vi "Address setting.vi"(7 "Address Cluster out输入":T1={"SPU"=refnum, "MPM"=[], "Port_Count"=0.0, "MPM_Count"=0.0, "SPU_Resource"=[], "USB_Resource"=[], "MPM_Communicater"="", "MPM_Count"=0.0, "MPM_Address"=[], "MPM_Portnumber"=[], "SPU_DeviveID"="", "MPM_communcation_method"=[], "TSL_sweepstartwave"=0.0, "TSL_sweepstopwave"=0.0, "TSL_Address"="", "TSL_Communicater"="", "TSL"=refnum, "tsl_communcation_method"=3, "TSL_Portnumber"=0.0} {"tsl_communcation_method" items=["GPIB", "C232C", "TCPIP", "USB"]; "MPM_communcation_method" items=["GPIB", "C232C", "TCPIP", "USB"]}, 8 "错误输入（无错误）":errorcluster caption="error in", 11 "SPU in":refnum<k24>) -> (0 "error out":errorcluster, 1 "Address Cluster out输出":T1={"SPU"=refnum, "MPM"=[], "Port_Count"=0.0, "MPM_Count"=0.0, "SPU_Resource"=[], "USB_Resource"=[], "MPM_Communicater"="", "MPM_Count"=0.0, "MPM_Address"=[], "MPM_Portnumber"=[], "SPU_DeviveID"="", "MPM_communcation_method"=[], "TSL_sweepstartwave"=0.0, "TSL_sweepstopwave"=0.0, "TSL_Address"="", "TSL_Communicater"="", "TSL"=refnum, "tsl_communcation_method"=3, "TSL_Portnumber"=0.0} {"tsl_communcation_method" items=["GPIB", "C232C", "TCPIP", "USB"]; "MPM_communcation_method" items=["GPIB", "C232C", "TCPIP", "USB"]})   [LabVIEW 2017]
doc: "'----Apply to communication parametere from Instrument setting form"
uses:
  CTL/Address Cluster.ctl
  D:/test/ILSTS/LV_IL_Sample/DLL/InstrumentDLL.dll
  DLL/InstrumentDLL.dll
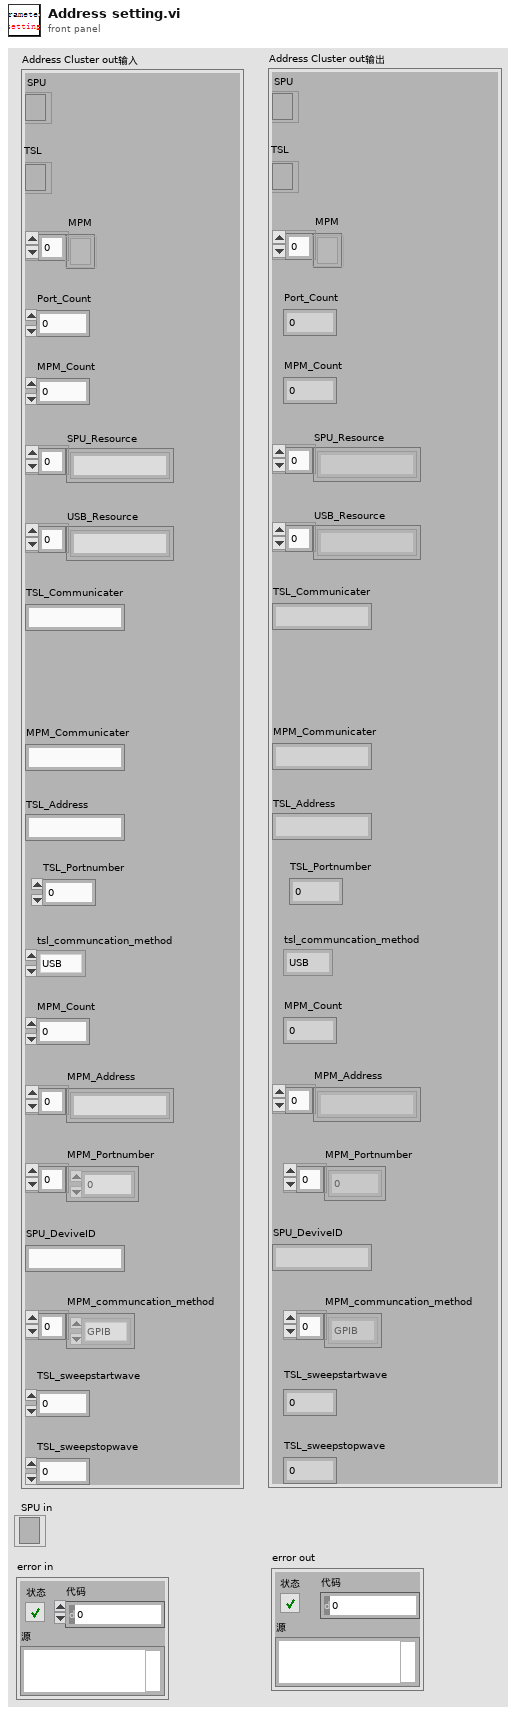
[diagram p1: front panel]
types:
  T1 = typedef "Address Cluster.ctl" = cluster{"SPU":refnum<k24>, "MPM":refnum<k24>[], "Port_Count":dbl, "MPM_Count":dbl, "SPU_Resource":string[], "USB_Resource":string[], "MPM_Communicater":string, "MPM_Count":dbl, "MPM_Address":string[], "MPM_Portnumber":dbl[], "SPU_DeviveID":string, "MPM_communcation_method":i32[], "TSL_sweepstartwave":dbl, "TSL_sweepstopwave":dbl, "TSL_Address":string, "TSL_Communicater":string, "TSL":refnum<k24>, "tsl_communcation_method":i32, "TSL_Portnumber":dbl}
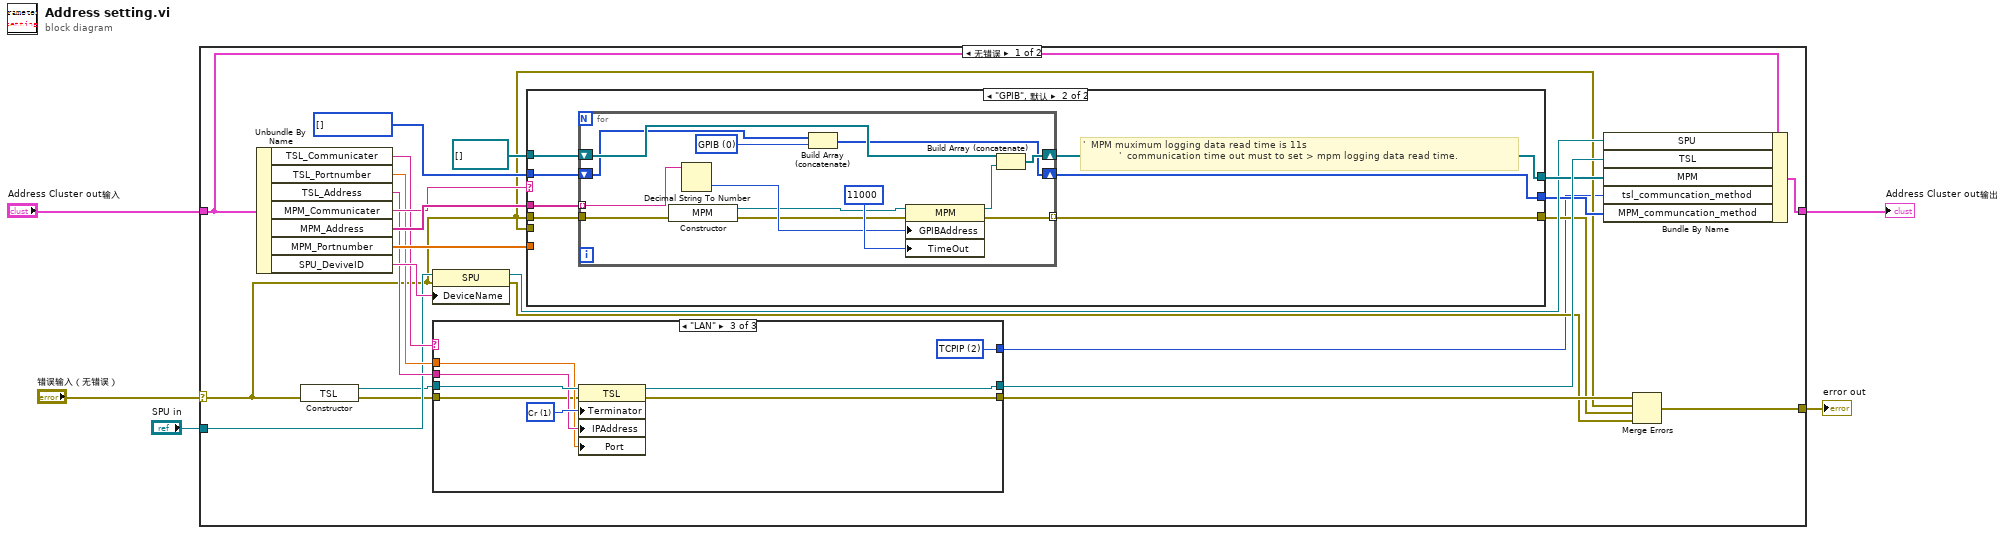
[diagram p0: block diagram]
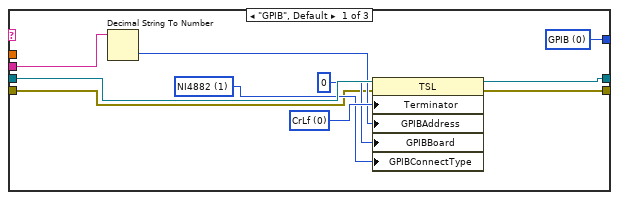
[diagram p2: hidden frame]
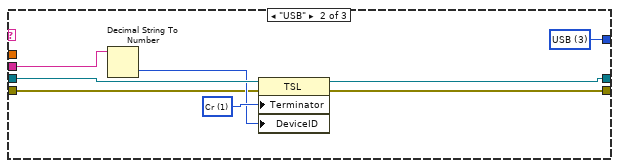
[diagram p3: hidden frame]
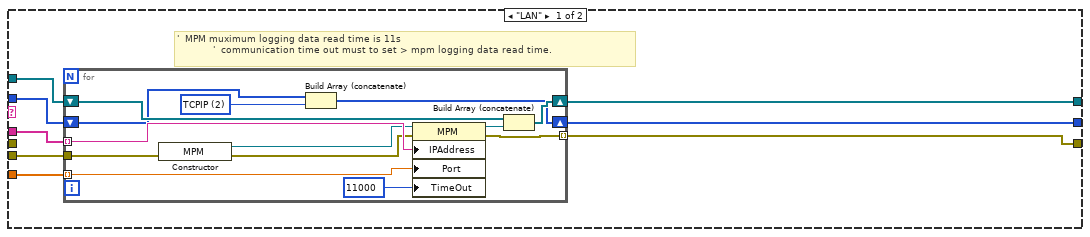
[diagram p4: hidden frame]
diagram:
  n1 = case shown="无错误" "错误输入（无错误）" {
    selector: "错误输入（无错误）" -> [w9 w98]
    tunnel: [w29 w97] -> w5
    tunnel: "Address Cluster out输入" -> [w25 w97]
    tunnel: [w11 w98] -> w3
    tunnel: "SPU in" -> [w10 _]
    frame No Error {
      w23 = i32[] [] items=["GPIB", "C232C", "TCPIP", "USB"] ("tsl_communcation_method")
      n2 = Unbundle By Name(w25) -> ("TSL_Communicater"=w16:string, "TSL_Portnumber"=w18:dbl, "TSL_Address"=w17:string, "MPM_Communicater"=w19:string, "MPM_Address"=w20:string[], "MPM_Portnumber"=w21:dbl[], "SPU_DeviveID"=w24:string)
      n3 = constructor class="TSL"(error in=w9) -> (reference out=w8:refnum<k24>, error out=w7:errorcluster)  [unwired: 2 in, 1 out]
      n4 = property on="属性节点" class="SPU"(reference=w10, error in=w9, "DeviceName"=w24) -> (reference out=w26:refnum<k24>, error out=w12:errorcluster)
      n5 = case shown="\"LAN\"" w16 {
        tunnel: w8 -> [w39 w47 w55]
        tunnel: [w30 w40 w48] -> w28
        tunnel: w17 -> [w37 w45 w53]
        tunnel: w18 -> [_ _ w52]
        tunnel: w7 -> [w33 w43 w51]
        tunnel: [w32 w42 w50] -> w14
        tunnel: [w31 w41 w49] -> w6
        frame "GPIB", Default {
          w34 = 1 items=["NIVisa", "NI4882", "KeysightIO"] ("GPIBConnectType")
          w38 = 0 items=["CrLf", "Cr", "Lf"] ("Terminator")
          w31 = 0 items=["GPIB", "C232C", "TCPIP", "USB"] ("method")
          n6 = Decimal String To Number(string=w37) -> (number=w36:i32)  [unwired: 2 in, 1 out]
          n7 = property on="属性节点" class="TSL"(reference=w39, error in=w33, "Terminator"=w38, "GPIBAddress"=w36, "GPIBBoard"=0, "GPIBConnectType"=w34) -> (reference out=w30:refnum<k24>, error out=w32:errorcluster)
        }
        frame "USB" {
          w46 = 1 items=["CrLf", "Cr", "Lf"] ("Terminator")
          w41 = 3 items=["GPIB", "C232C", "TCPIP", "USB"] ("method")
          n8 = Decimal String To Number(string=w45) -> (number=w44:i32)  [unwired: 2 in, 1 out]
          n9 = property on="属性节点" class="TSL"(reference=w47, error in=w43, "Terminator"=w46, "DeviceID"=w44) -> (reference out=w40:refnum<k24>, error out=w42:errorcluster)
        }
        frame "LAN" {
          w54 = 1 items=["CrLf", "Cr", "Lf"] ("Terminator")
          w49 = 2 items=["GPIB", "C232C", "TCPIP", "USB"] ("method")
          n10 = property on="属性节点" class="TSL"(reference=w55, error in=w51, "Terminator"=w54, "IPAddress"=w53, "Port"=w52) -> (reference out=w48:refnum<k24>, error out=w50:errorcluster)
        }
      }
      n11 = case shown="\"GPIB\", 默认" w19 {
        tunnel: w20 -> [w63 w83]
        tunnel: w21 -> [w62 _]
        tunnel: refnum<k24>[] [] ("添加的数组") -> [w61 w82]
        tunnel: w23 -> [w60 w81]
        tunnel: [w59 w80] -> w27
        tunnel: [w58 w79] -> w15
        tunnel: [w57 w78] -> w13
        tunnel: w9 -> [_ w77]
        tunnel: w9 -> [w56 _]
        frame "LAN" {
          # "'  MPM muximum logging data read time is 11s\n            '  communication time out must to set > mpm logging data read time."
          n12 = for {
            shift-right: [w72] -> w59
            shift-left: w61 -> [w73]
            tunnel: w63 -> [w76] mode=indexing
            tunnel: w62 -> [w75] mode=indexing
            shift-right: [w69] -> w58
            shift-left: w60 -> [w71]
            tunnel: [w67] -> w57 mode=indexing
            tunnel: w56 -> [w66]
            w70 = 2 items=["GPIB", "C232C", "TCPIP", "USB"] ("method")
            n13 = constructor class="MPM"(error in=w66) -> (reference out=w65:refnum<k24>, error out=w64:errorcluster)  [unwired: 2 in, 1 out]
            n14 = Build Array (concatenate)(w71, w70) -> (w69:i32[])
            n15 = property on="属性节点" class="MPM"(reference=w65, error in=w64, "IPAddress"=w76, "Port"=w75, "TimeOut"=11000) -> (reference out=w74:refnum<k24>, error out=w67:errorcluster)
            n16 = Build Array (concatenate)(w73, w74) -> (w72:refnum<k24>[])
          }
        }
        frame "GPIB", Default {
          # "'  MPM muximum logging data read time is 11s\n            '  communication time out must to set > mpm logging data read time."
          n17 = for {
            shift-right: [w94] -> w80
            shift-left: w82 -> [w95]
            tunnel: w83 -> [w90] mode=indexing
            shift-right: [w91] -> w79
            shift-left: w81 -> [w93]
            tunnel: [w88] -> w78 mode=indexing
            tunnel: w77 -> [w84]
            w92 = 0 items=["GPIB", "C232C", "TCPIP", "USB"] ("method")
            n18 = constructor class="MPM"(error in=w84) -> (reference out=w86:refnum<k24>, error out=w85:errorcluster)  [unwired: 2 in, 1 out]
            n19 = Decimal String To Number(string=w90) -> (number=w87:i32)  [unwired: 2 in, 1 out]
            n20 = Build Array (concatenate)(w93, w92) -> (w91:i32[])
            n21 = property on="属性节点" class="MPM"(reference=w86, error in=w85, "GPIBAddress"=w87, "TimeOut"=11000) -> (reference out=w96:refnum<k24>, error out=w88:errorcluster)
            n22 = Build Array (concatenate)(w95, w96) -> (w94:refnum<k24>[])
          }
        }
      }
      n23 = Bundle By Name(cluster=w25, "SPU"=w26, "TSL"=w28, "MPM"=w27, "tsl_communcation_method"=w6, "MPM_communcation_method"=w15) -> (w29:T1)
      n24 = Merge Errors(w14, w9, w13, w12) -> (w11:errorcluster)
    }
    frame Error {
    }
  }
  "Address Cluster out输出" <- w5
  "error out" <- w3
